vi "Build Project Tree Menu.vi"(9 "Coords":T1, 10 "Project Tree Menu":refnum<k9>, 11 "Project Tree":refnum<vi>) -> (3 "Discard":bool)   [LabVIEW 2015, in "Editor.lvclass"]
uses:
  Editor.lvclass
  <vilib>/Utility/miscctls.llb/LVPoint32TypeDef.ctl
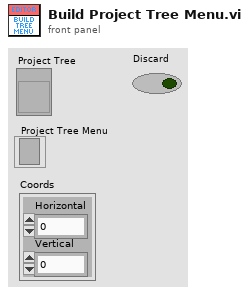
[diagram p1: front panel]
types:
  T1 = typedef "LVPoint32TypeDef.ctl" = cluster{"Horizontal":i32, "Vertical":i32}
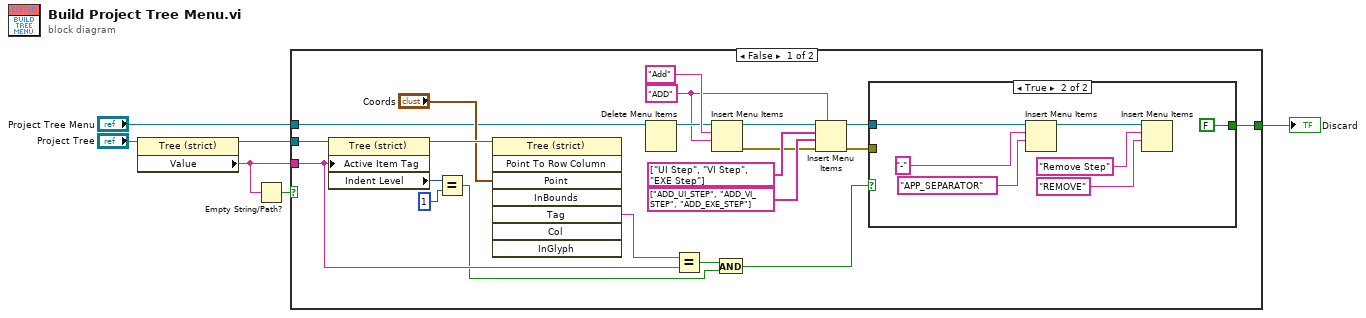
[diagram p0: block diagram]
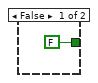
[diagram p2: hidden frame]
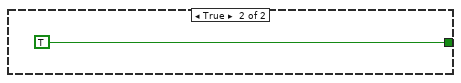
[diagram p3: hidden frame]
diagram:
  n1 = property class="Tree (strict)"(reference="Project Tree") -> (reference out=w6:refnum<vi>, "Value"=w5:string)  [unwired: 1 in, 1 out]
  n2 = Empty String/Path?(string/path=w5) -> (empty?=w4:bool)
  n3 = case shown="False" w4 {
    tunnel: w6 -> [w27 _]
    tunnel: w5 -> [w20 _]
    tunnel: "Project Tree Menu" -> [w16 _]
    tunnel: [w24 TRUE] -> w2
    frame False {
      w12 = "ADD"
      n4 = property class="Tree (strict)"(reference=w27, "Active Item Tag"=w20) -> (reference out=w23:refnum<vi>, "Indent Level"=w26:i32)  [unwired: 1 in, 1 out]
      n5 = Equal?(x=w26, y=1) -> (x = y?=w18:bool)
      n6 = invoke class="Tree (strict)" method="Point To Row Column"(reference=w23, "Point"="Coords") -> ("Tag"=w21:string)  [unwired: 6 in, 7 out]
      n7 = Delete Menu Items(9:w16) -> (3:w14:refnum<k9>)  [unwired: 3 in, 1 out]
      n8 = Equal?(x=w21, y=w20) -> (x = y?=w19:bool)
      n9 = Insert Menu Items(7:w12, 8:"Add", 9:w14) -> (0:w8:errorcluster, 3:w11:refnum<k9>)  [unwired: 3 in, 1 out]
      n10 = And(x=w19, y=w18) -> (x .and. y?=w17:bool)
      n11 = Insert Menu Items(5:w12, 6:w8, 7:string[] ["ADD_UI_STEP", "ADD_VI_STEP", "ADD_EXE_STEP"], 8:string[] ["UI Step", "VI Step", "EXE Step"], 9:w11) -> (0:w7:errorcluster, 3:w13:refnum<k9>)  [unwired: 1 in, 1 out]
      n12 = case shown="True" w17 {
        tunnel: w13 -> [_ w30]
        tunnel: [FALSE FALSE] -> w24
        tunnel: w7 -> [_ _]
        frame False {
        }
        frame True {
          n13 = Insert Menu Items(7:"APP_SEPARATOR" ("menu tag"), 8:"-", 9:w30) -> (3:w29:refnum<k9>)  [unwired: 3 in, 2 out]
          n14 = Insert Menu Items(7:"REMOVE" ("menu tag"), 8:"Remove Step", 9:w29) -> ()  [unwired: 3 in, 3 out]
        }
      }
    }
    frame True {
    }
  }
  "Discard" <- w2
